vi "Controller Enqeuer FGV.vi"(7 "State":enum16{"Store", "Send MSG"}(ring)=enum."Send MSG", 10 "MSG":refnum<class "Message.lvclass">, 11 "Enqueuer":refnum<class "Message Enqueuer.lvclass">) -> (0 "error out":errorcluster)   [LabVIEW 2014, in "Controller.lvlib" / "Controller.lvclass"]
doc: "This is a functional global variable for facillitating communication between web services and the main controller. This allows the web services to enqueue messages to be handled by the controller directly by the web service itself."
uses:
  Controller.lvclass
  <vilib>/ActorFramework/Message Enqueuer/Message Enqueuer.lvclass
  <vilib>/ActorFramework/Message/Message.lvclass
  <vilib>/ActorFramework/Message Enqueuer/Message Enqueuer.lvclass/Message Enqueuer.ctl
  <vilib>/ActorFramework/Message Priority Queue/Priority Enqueue.vi
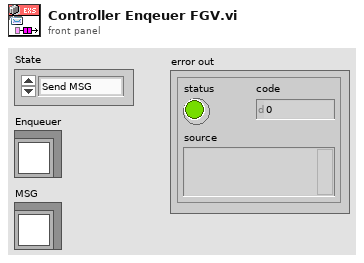
[diagram p1: front panel]
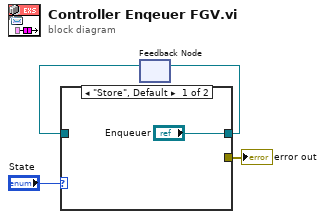
[diagram p0: block diagram]
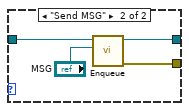
[diagram p2: hidden frame]
diagram:
  n1 = feedback #1() -> (w2:refnum<class "Message Enqueuer.lvclass">)  [unwired: 1 in]
  n2 = case shown="\"Store\", Default" "State" {
    tunnel: w2 -> [_ w9]
    tunnel: ["Enqueuer" w8] -> w3
    tunnel: [_ w7] -> w1
    frame "Store", Default {
    }
    frame "Send MSG" {
      n3 = call <vilib>:"Enqueue.vi"("Message"="MSG", "Message Enqueuer in"=w9) -> ("error out"=w7:errorcluster, "Message Enqueuer out"=w8:refnum<class "Message Enqueuer.lvclass">)  [unwired: 8 in]
    }
  }
  "error out" <- w1
  n4 = feedback-in #1(w3) -> ()
